vi "Create Instrument Addon_ex.vi"() -> ()   [LabVIEW 2019]
uses:
  NationalInstruments.VeriStand.SystemDefinitionAPI
  Addon/Support Libraries/Protocols.lvlibp/TCP/TCP.lvclass
  <vilib>/NI VeriStand/Custom Device API/Custom Device Item Ref.ctl
  Scripting API/Scripting API.lvlib
  <vilib>/NI VeriStand/Custom Device API/Custom Device API.lvlib
panel:
  out "Target Out":refnum<k24>
  out "Instrument Addon Refnum":T1=18446744073709551615 format="%.0x"
  out "Message Channels Refnums":T2 {"Enable Periodic" format="%.0x"; "Error Code" format="%.0x"; "Message Status" format="%.0x"; "Timestamp" format="%.0x"; "Trigger" format="%.0x"}
  out "Error Out":errorcluster
  in  "Protocol In":refnum<class "TCP.lvclass">
  in  "PCL Decimation":u16
  in  "Error In":errorcluster
  in  "Target In":refnum<k24>
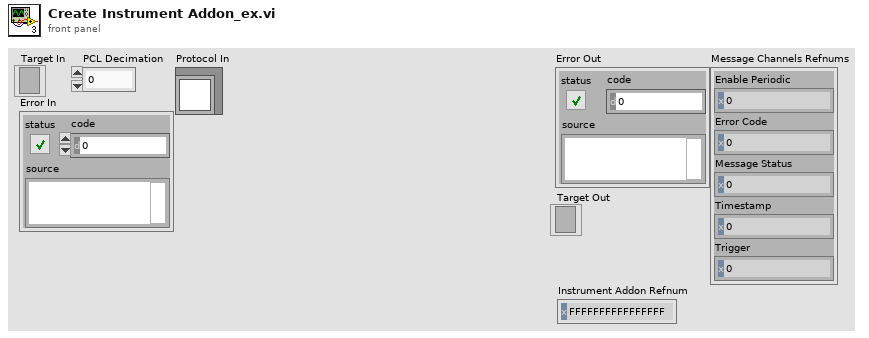
[diagram p1: front panel]
types:
  T1 = typedef "Custom Device API.lvlib/Custom Device Item Ref.ctl" = u64
  T2 = cluster{"Enable Periodic":T1, "Error Code":T1, "Message Status":T1, "Timestamp":T1, "Trigger":T1}
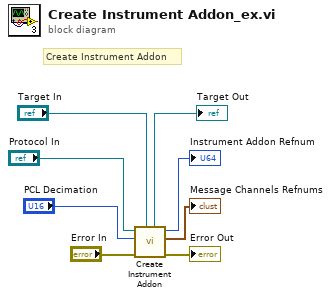
[diagram p0: block diagram]
diagram:
  # "Create Instrument Addon"
  n1 = call "Create Instrument Addon.vi"("Target In"="Target In", "Error In"="Error In", "PCL Decimation"="PCL Decimation", "Protocol In"="Protocol In") -> ("Error Out"=→"Error Out":errorcluster, "Message Channels Refnums"=→"Message Channels Refnums":T2, "Instrument Addon Refnum"=→"Instrument Addon Refnum":T1, "Target Out"=→"Target Out":refnum<k24>)  [unwired: 4 in]
